vi "wavelenghtToindex.vi"(10 "WL in":dbl, 11 "WL Values":dbl[](array[numeric])) -> (3 "index of WL":i32)   [LabVIEW 2021]
doc: "Random Laser Project\nAndré Romero - 2020\nandretec@ifsc.usp.br\n\nConvert Wavelenght to index of table WL"
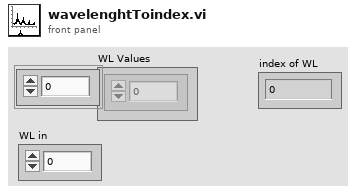
[diagram p1: front panel]
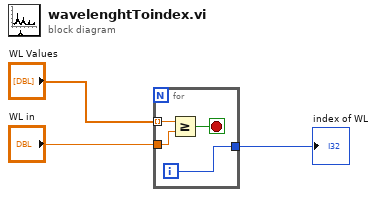
[diagram p0: block diagram]
diagram:
  n1 = for {
    tunnel: "WL Values" -> [w7] mode=indexing
    tunnel: "WL in" -> [w6]
    tunnel: [w4] -> w1
    i -> [w4]
    stop <- w5 stop-if-true
    n2 = Greater Or Equal?(x=w7, y=w6) -> (x >= y?=w5:bool)
  }
  "index of WL" <- w1
